vi "string_to_long_int.vi"(8 "error in (no error)":errorcluster, 10 "Long (string)":string) -> (0 "error out":errorcluster, 2 "Long (int)":i64)   [LabVIEW 2018, in "Inficon IC6.lvlib"]
doc: "Convert an IC6 response string representing a signed long integer into a LabVIEW I64."
uses:
  <instrlib>/Inficon IC6/Inficon IC6.lvlib
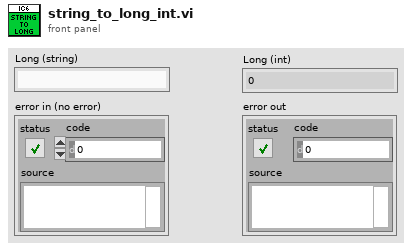
[diagram p1: front panel]
types:
  T1 = enum16{"big-endian, network order", "native, host order", "little-endian"}
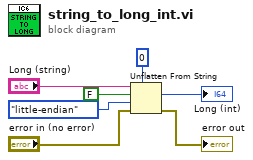
[diagram p0: block diagram]
diagram:
  n1 = Unflatten From String(type=i64 0 ("offset (0)"), binary string="Long (string)", data includes array or string size? (T)=FALSE, byte order (0:big-endian, network order)=T1."little-endian", error in (no error)="error in (no error)") -> (value=→"Long (int)":i64, error out=→"error out":errorcluster)  [unwired: 1 out]
